vi "init_instruments.vi"(6 "Lock-in resource name":refnum<visa-resource-name>="GPIB1::8::INSTR", 7 "PSU resource name":refnum<visa-resource-name>="COM6", 9 "Input Connection (0: Single-Ended Voltage)":u16(ring) items=["Single-Ended Voltage", "Differential Voltage", "1 MOhm Current Gain", "100 MOhm Current Gain"], 10 "Monochromator Addr in":string) -> (0 "LED power supply":bool, 1 "Pixel Selector":bool, 3 "Monochromator":bool, 4 "Lock-in amplifier":bool)   [LabVIEW 2018]
uses:
  <vilib>/Instr/_visa.llb/VISA Configure Serial Port (Instr).vi
panel:
  out "TTi power supply":refnum<visa-resource-name>
  out "SR830":refnum<visa-resource-name>
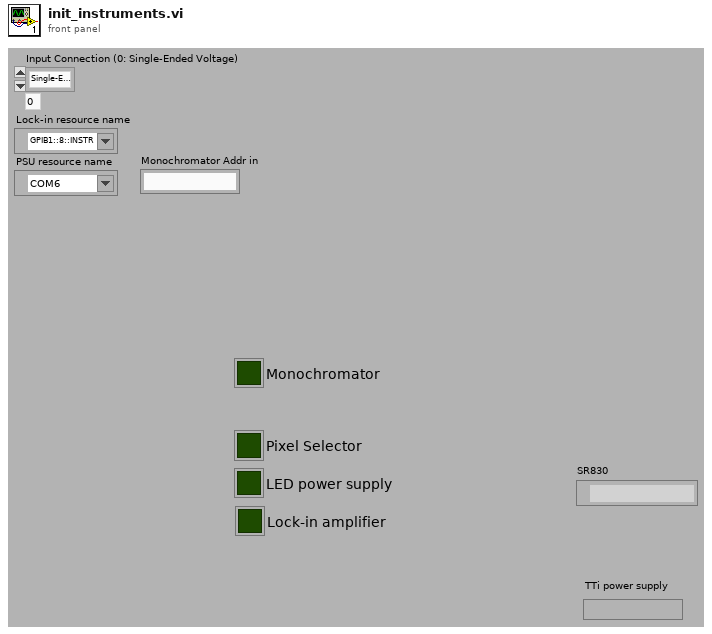
[diagram p1: front panel]
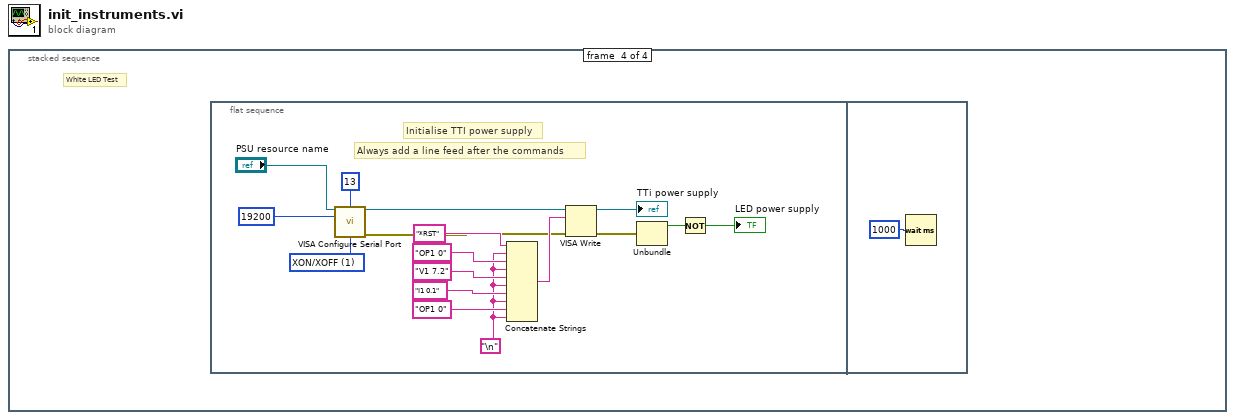
[diagram p0: block diagram]
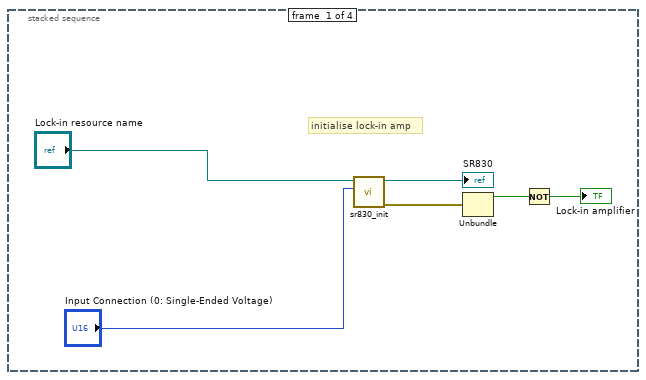
[diagram p2: hidden frame]
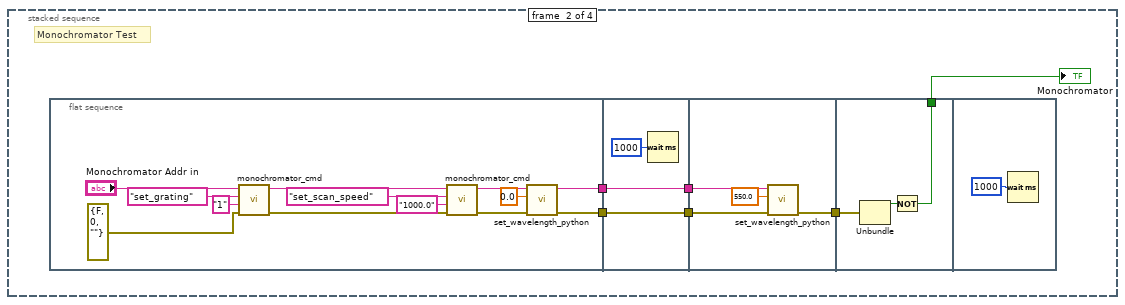
[diagram p3: hidden frame]
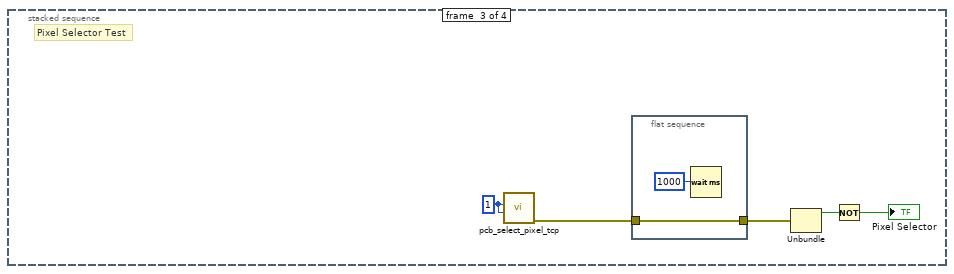
[diagram p4: hidden frame]
diagram:
  n1 = stacked-sequence {
    frame #0 {
      # "initialise lock-in amp"
      n2 = call "sr830_init.vi"("Input Connection (0: Single-Ended Voltage)"="Input Connection (0: Single-Ended Voltage)", "VISA resource name"="Lock-in resource name") -> ("error out"=w5:errorcluster, "SR830"=→"SR830":refnum<visa-resource-name>)  [unwired: 4 in]
      n3 = Unbundle(w5) -> ("status"=w4:bool)  [unwired: 2 out]
      n4 = Not(x=w4) -> (.not. x?=→"Lock-in amplifier":bool)
    }
    frame #1 {
      # "Monochromator Test"
      n5 = flat-sequence {
        tunnel: [w15] -> w11
        tunnel: [w14] -> w7
        tunnel: [w27] -> w12
        tunnel: w11 -> [w27]
        tunnel: [w26] -> w8
        tunnel: w7 -> [w26]
        tunnel: w12 -> [w30]
        tunnel: [w29] -> w10
        tunnel: w8 -> [w31]
        tunnel: w10 -> [w35]
        tunnel: [w33] -> w9
        frame #0 {
          n6 = call "monochromator_cmd.vi"("error in (no error)"=errorcluster {"status"=FALSE, "code"=0, "source"=""} ("error constant"), "Parameter"="1", "Command"="set_grating", "Addr in"="Monochromator Addr in") -> ("error out"=w25:errorcluster, "Addr out"=w24:string)  [unwired: 4 in, 2 out]
          n7 = call "monochromator_cmd.vi"("error in (no error)"=w25, "Parameter"="1000.0", "Command"="set_scan_speed", "Addr in"=w24) -> ("error out"=w17:errorcluster, "Addr out"=w18:string)  [unwired: 4 in, 2 out]
          n8 = call "set_wavelength_python.vi"("error in (no error)"=w17, "wavelength"=0.0, "Addr"=w18) -> ("error out"=w15:errorcluster, "Addr out"=w14:string)  [unwired: 7 in]
        }
        frame #1 {
          n9 = Wait (ms)(milliseconds to wait=i16 1000 ("Spectrometer Handle in")) -> ()  [unwired: 1 out]
        }
        frame #2 {
          n10 = call "set_wavelength_python.vi"("error in (no error)"=w30, "wavelength"=550.0, "Addr"=w31) -> ("error out"=w29:errorcluster)  [unwired: 7 in, 1 out]
        }
        frame #3 {
          n11 = Unbundle(w35) -> ("status"=w34:bool)  [unwired: 2 out]
          n12 = Not(x=w34) -> (.not. x?=w33:bool)
        }
        frame #4 {
          n13 = Wait (ms)(milliseconds to wait=i16 1000 ("Spectrometer Handle in")) -> ()  [unwired: 1 out]
        }
      }
      "Monochromator" <- w9
    }
    frame #2 {
      w41 = u32 1 ("Pixel")
      # "Pixel Selector Test"
      n14 = call "pcb_select_pixel_tcp.vi"("Cell"=w41, "Pixel"=w41) -> ("error out"=w40:errorcluster)  [unwired: 8 in, 1 out]
      n15 = flat-sequence {
        tunnel: w40 -> [w42]
        tunnel: [w42] -> w39
        frame #0 {
          n16 = Wait (ms)(milliseconds to wait=i16 1000 ("Spectrometer Handle in")) -> ()  [unwired: 1 out]
        }
      }
      n17 = Unbundle(w39) -> ("status"=w38:bool)  [unwired: 2 out]
      n18 = Not(x=w38) -> (.not. x?=→"Pixel Selector":bool)
    }
    frame #3 {
      # "White LED Test"
      n19 = flat-sequence {
        frame #0 {
          w49 = "\n"
          w56 = u16 1 items=["None", "XON/XOFF", "RTS/CTS", "XON/XOFF & RTS/CTS", "DTR/DSR", "XON/XOFF & DTR/DSR"] ("flow control (0:none)")
          # "Initialise TTI power supply"
          # "Always add a line feed after the commands"
          n20 = call-poly "VISA Configure Serial Port"("VISA resource name"="PSU resource name", "termination char\n(0xA = '\\n' = LF)"=u8 13 ("termination char\n(0xA = '\\n' = LF)"), "baud rate (9600)"=u32 19200, "flow control (0:none)"=w56) -> ("VISA resource name out"=w47:refnum<visa-resource-name>, "error out"=w44:errorcluster)  [unwired: 10 in]
          n21 = Concatenate Strings("*RST" ("string"), w49, "OP1 0" ("string"), w49, "V1 7.2" ("string"), w49, "I1 0.1" ("string"), w49, "OP1 0" ("string"), w49) -> (w48:string)
          n22 = VISA Write(VISA resource name=w47, write buffer=w48, error in (no error)=w44) -> (VISA resource name out=→"TTi power supply":refnum<visa-resource-name>, error out=w60:errorcluster)  [unwired: 1 out]
          n23 = Unbundle(w60) -> ("status"=w45:bool)  [unwired: 2 out]
          n24 = Not(x=w45) -> (.not. x?=→"LED power supply":bool)
        }
        frame #1 {
          n25 = Wait (ms)(milliseconds to wait=i16 1000 ("Spectrometer Handle in")) -> ()  [unwired: 1 out]
        }
      }
    }
  }
